vi "Untitled 1.vi"() -> ()   [LabVIEW 2017]
panel:
  out "Array 7":u32[](array[numeric])=[97, 99, 101, 103, 105, 107, 109, 111, 145, 147, 149, 151, 153, 155, 157, 159, 193, 195, 197, 199, 201, 203, 205, 207, 241, 243, 245, 247, 249, 251, 253, 255] format="%x"
  out "Array 6":u32[](array[numeric])=[97, 99, 101, 103, 105, 107, 109, 111, 145, 147, 149, 151, 153, 155, 157, 159, 193, 195, 197, 199, 201, 203, 205, 207, 241, 243, 245, 247, 249, 251, 253, 255] format="%x"
  in  "Thresholds":u16=600
  in  "one key for threshold":bool
  in  "SMA mode":bool
  in  "Thresholds (mV)":u16[](array[numeric])=[580, 580, 600, 600, 600, 600, 600, 600, 580, 580, 600, 600, 600, 600, 600, 600, 580, 580, 600, 600, 600, 600, 600, 600, 580, 580, 600, 600, 600, 600, 600, 600]
  out "Array":u32[](array[numeric])=[96, 98, 100, 102, 104, 106, 108, 110, 144, 146, 148, 150, 152, 154, 156, 158, 192, 194, 196, 198, 200, 202, 204, 206, 240, 242, 244, 246, 248, 250, 252, 254] format="%x"
  out "Array 2":u32[](array[numeric])=[97, 99, 101, 103, 105, 107, 109, 111, 145, 147, 149, 151, 153, 155, 157, 159, 193, 195, 197, 199, 201, 203, 205, 207, 241, 243, 245, 247, 249, 251, 253, 255] format="%x"
  out "Array 3":u32[](array[numeric])=[96, 98, 100, 102, 104, 106, 108, 110, 144, 146, 148, 150, 152, 154, 156, 158, 192, 194, 196, 198, 200, 202, 204, 206, 240, 242, 244, 246, 248, 250, 252, 254] format="%x"
  out "Array 4":u32[](array[numeric])=[96, 98, 100, 102, 104, 106, 108, 110, 144, 146, 148, 150, 152, 154, 156, 158, 192, 194, 196, 198, 200, 202, 204, 206, 240, 242, 244, 246, 248, 250, 252, 254] format="%x"
  out "Array 5":u32[](array[numeric])=[97, 99, 101, 103, 105, 107, 109, 111, 145, 147, 149, 151, 153, 155, 157, 159, 193, 195, 197, 199, 201, 203, 205, 207, 241, 243, 245, 247, 249, 251, 253, 255] format="%x"
  in  "address":string="192.168.10.10"
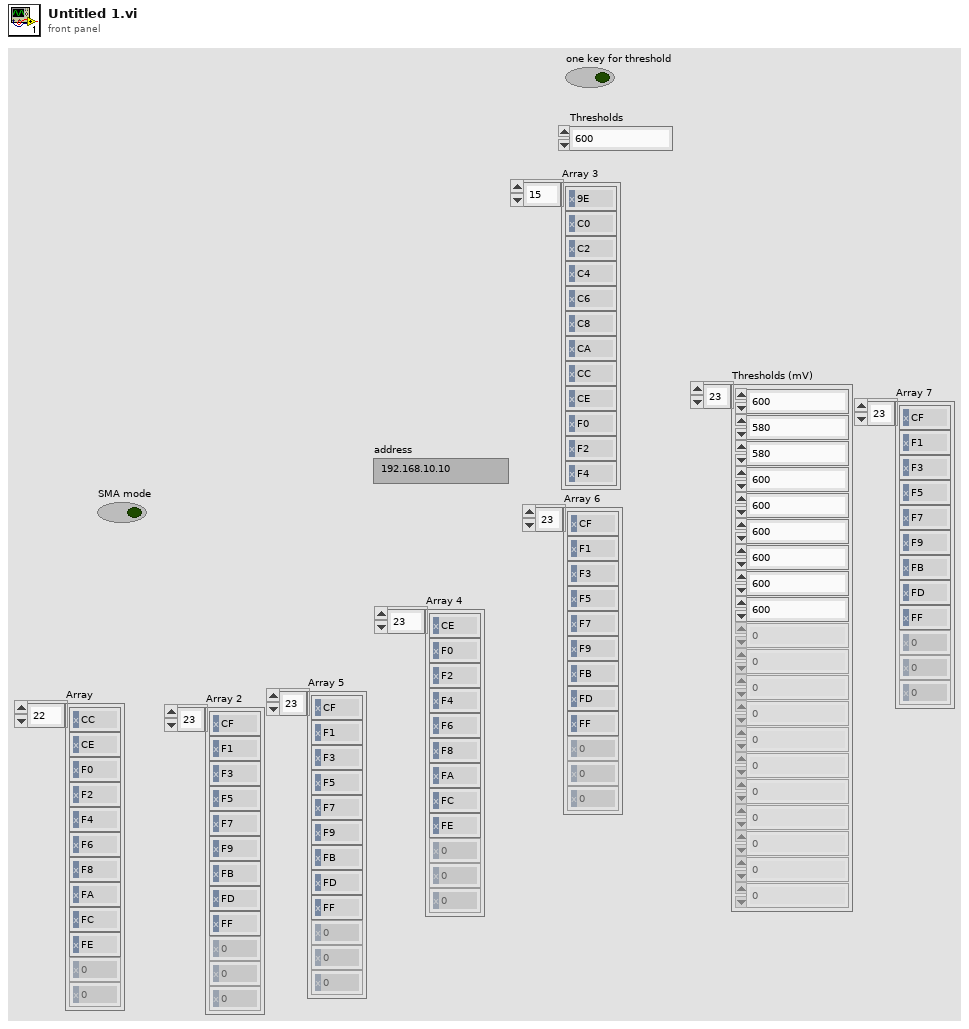
[diagram p1: front panel]
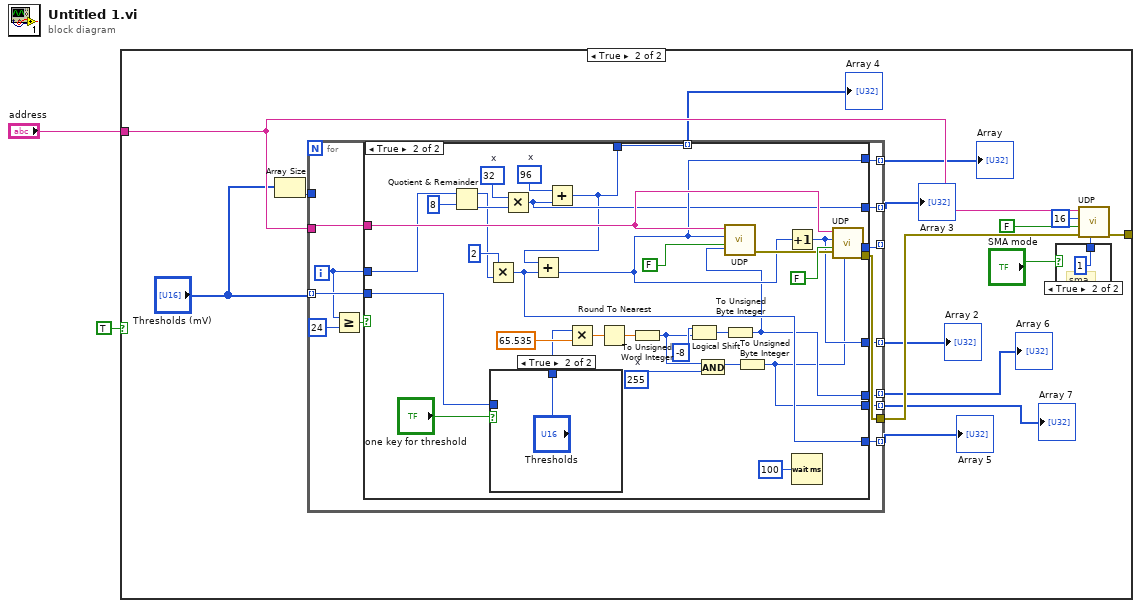
[diagram p0: block diagram]
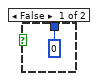
[diagram p3: hidden frame]
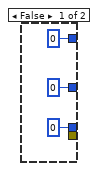
[diagram p4: hidden frame]
diagram:
  n1 = case shown="True" TRUE {
    tunnel: "address" -> [_ w18]
    tunnel: [_ w15] -> _
    frame False {
    }
    frame True {
      n2 = Array Size(array="Thresholds (mV)") -> (size(s)=w11:i32)
      n3 = for {
        tunnel: w18 -> [w34]
        tunnel: "Thresholds (mV)" -> [w26] mode=indexing
        tunnel: [w33] -> _ mode=indexing
        tunnel: [w32] -> w16
        tunnel: w11 -> [_]
        tunnel: [w31] -> w9 mode=indexing
        tunnel: [w30] -> w8 mode=indexing
        tunnel: [w29] -> w7 mode=indexing
        tunnel: [w28] -> w6 mode=indexing
        tunnel: [w27] -> w5 mode=indexing
        tunnel: [w22] -> w4 mode=indexing
        tunnel: [w21] -> w3 mode=indexing
        i -> [w25]
        n4 = Greater Or Equal?(x=w25, y=24) -> (x >= y?=w23:bool)
        n5 = case shown="True" w23 {
          tunnel: w34 -> [_ w64]
          tunnel: [u8 0 ("Out") w59] -> w33
          tunnel: [_ w55] -> w32
          tunnel: w26 -> [_ w52]
          tunnel: w25 -> [_ w47]
          tunnel: [0 w46] -> w31
          tunnel: [_ w45] -> w30
          tunnel: [0 w44] -> w29
          tunnel: [_ w43] -> w28
          tunnel: [_ w42] -> w27
          tunnel: [_ w39] -> w22
          tunnel: [_ w38] -> w21
          frame False {
          }
          frame True {
            w48 = u16 96  # x
            w49 = u16 32  # x
            w61 = u16 255  # x
            n6 = Quotient & Remainder(x=w47, y=8) -> (x-y*floor(x/y)=w41:i32, floor(x/y)=w50:i32)
            n7 = Multiply(x=2, y=w41) -> (x*y=w42:i32)
            n8 = case shown="True" "one key for threshold" {
              tunnel: [w70 "Thresholds"] -> w53
              tunnel: w52 -> [w70 _]
              frame False {
              }
              frame True {
              }
            }
            n9 = Multiply(x=w49, y=w50) -> (x*y=w44:i32)
            n10 = Add(x=w48, y=w44) -> (x+y=w43:i32)
            n11 = Add(x=w43, y=w42) -> (x+y=w46:i32)
            n12 = Multiply(x=w53, y=65.535) -> (x*y=w67:dbl)
            n13 = Round To Nearest(number=w67) -> (nearest integer value=w65:dbl)
            n14 = To Unsigned Word Integer(number=w65) -> (unsigned 16bit integer=w57:u16)
            n15 = Logical Shift(y=i16 -8, x=w57) -> (x << y=w62:u16)
            n16 = And(x=w57, y=w61) -> (x .and. y?=w60:u16)
            n17 = To Unsigned Byte Integer(number=w62) -> (unsigned 8bit integer=w39:u8)
            n18 = call "UDP.vi"("In"=w39, "Read (TRUE)"=FALSE, "Address"=w46, "IP address"=w64) -> ("error out"=w56:errorcluster)  [unwired: 5 in, 1 out]
            n19 = To Unsigned Byte Integer(number=w60) -> (unsigned 8bit integer=w38:u8)
            n20 = Increment(x=w46) -> (x+1=w45:i32)
            n21 = Wait (ms)(milliseconds to wait=u32 100) -> ()  [unwired: 1 out]
            n22 = call "UDP.vi"("In"=w38, "error in (no error)"=w56, "Read (TRUE)"=FALSE, "Address"=w45, "IP address"=w64) -> ("error out"=w55:errorcluster, "Out"=w59:u8)  [unwired: 4 in]
          }
        }
      }
      "Array" <- w9
      "Array 2" <- w8
      "Array 3" <- w7
      "Array 4" <- w6
      "Array 5" <- w5
      "Array 6" <- w4
      "Array 7" <- w3
      n23 = case shown="True" "SMA mode" {
        tunnel: [u8 0 ("In") u8 1 ("In")] -> w14
        frame False {
        }
        frame True {
          # "sma"
        }
      }
      n24 = call "UDP.vi"("In"=w14, "error in (no error)"=w16, "Read (TRUE)"=FALSE, "Address"=u32 16, "IP address"=w18) -> ("error out"=w15:errorcluster)  [unwired: 4 in, 1 out]
    }
  }
